vi "TESTE.vi"() -> ()   [LabVIEW 2018]
panel:
  out "number":i32
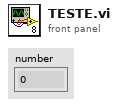
[diagram p1: front panel]
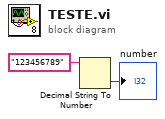
[diagram p0: block diagram]
diagram:
  n1 = Decimal String To Number(string="123456789") -> (number=→"number":i32)  [unwired: 2 in, 1 out]
